vi "FFConstVI-Working.vi"(8 "nXForce":i32(slide) scale=-10000.0..10000.0, 11 "millisecond multiple":u32) -> ()   [LabVIEW 2013]
uses:
  FFConstdll/FFConstDll.dll
  user32.dll
panel:
  out "Acquire HRESULT":i32
  out "Current ForegroundWindow HWND":u32
  out "Start ForegroundWindow HWND":u32
  in  "stop":bool
  out "SetDeviceForce HRESULT":i32
  out "Init HRESULT":i32
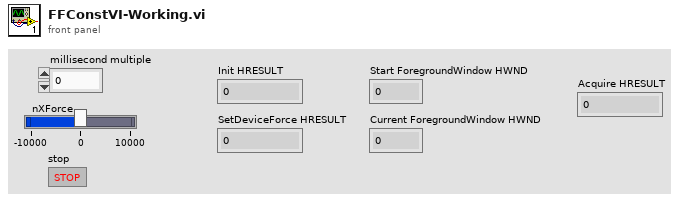
[diagram p1: front panel]
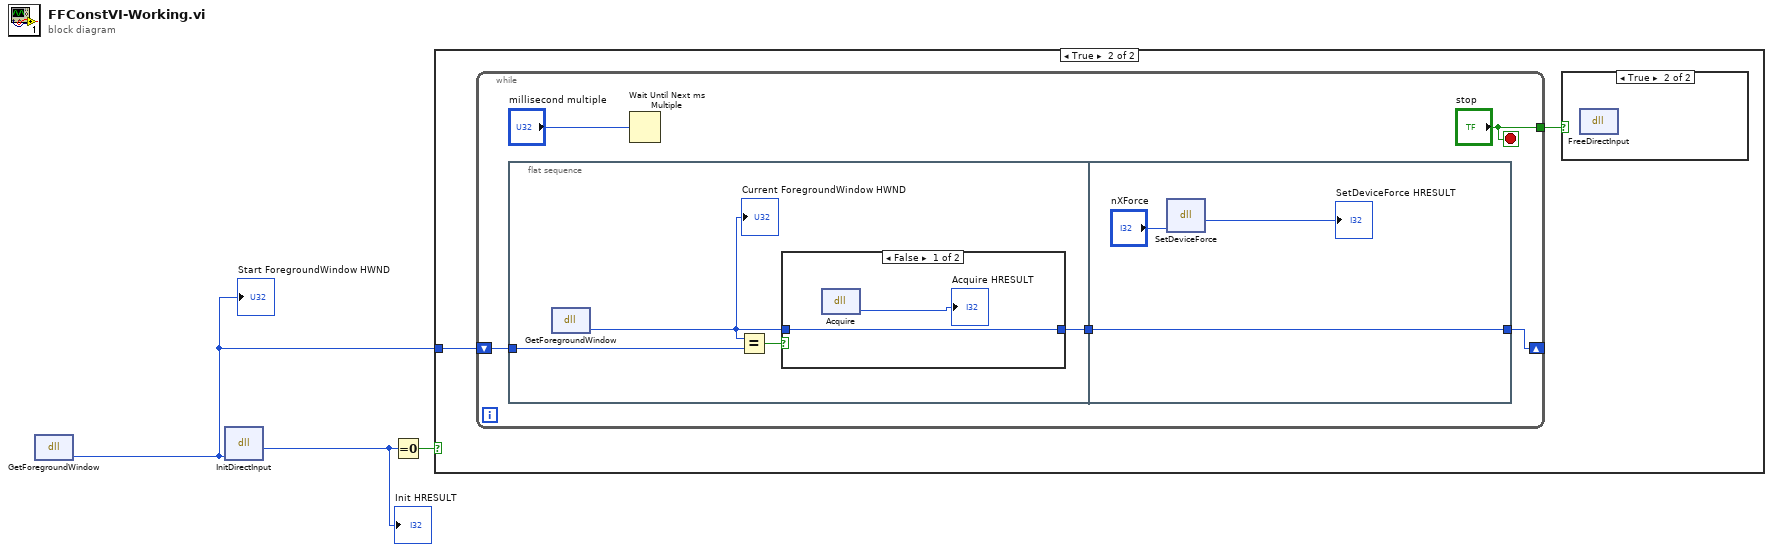
[diagram p0: block diagram]
diagram:
  n1 = dll-call lib="user32.dll" fn="GetForegroundWindow"() -> ("HWND"=w2:u32)  [unwired: 3 in, 2 out]
  "Start ForegroundWindow HWND" <- w2
  n2 = dll-call lib="C:/Users/user/Documents/Dropbox/Kettering/Robotics Team/RC Car Race Information/Teleop Labview Code/Winter '14 Force Feedback Experiment/FFConstdll/FFConstDll.dll" fn="InitDirectInput"("hDlg"=w2) -> ("HRESULT"=w1:u32)  [unwired: 4 in, 2 out]
  "Init HRESULT" <- w1
  n3 = Equal To 0?(x=w1) -> (x = 0?=w3:bool)
  n4 = case shown="True" w3 {
    tunnel: w2 -> [_ w4]
    frame False {
    }
    frame True {
      n5 = while {
        tunnel: ["stop"] -> w5
        shift-right: [w9] -> _
        shift-left: w4 -> [w7]
        stop <- "stop" stop-if-true
        n6 = flat-sequence {
          tunnel: w7 -> [w14]
          tunnel: [w11] -> w8
          tunnel: [w18] -> w9
          tunnel: w8 -> [w18]
          frame #0 {
            n7 = dll-call lib="user32.dll" fn="GetForegroundWindow"() -> ("HWND"=w12:u32)  [unwired: 3 in, 2 out]
            "Current ForegroundWindow HWND" <- w12
            n8 = Equal?(x=w12, y=w14) -> (x = y?=w13:bool)
            n9 = case shown="False" w13 {
              tunnel: w12 -> [w15 w17]
              tunnel: [w15 w17] -> w11
              frame False {
                n10 = dll-call lib="C:/Users/user/Documents/Dropbox/Kettering/Robotics Team/RC Car Race Information/Teleop Labview Code/Winter '14 Force Feedback Experiment/FFConstdll/FFConstDll.dll" fn="Acquire"() -> ("HRESULT"=→"Acquire HRESULT":i32)  [unwired: 3 in, 2 out]
              }
              frame True {
              }
            }
          }
          frame #1 {
            n11 = dll-call lib="C:/Users/user/Documents/Dropbox/Kettering/Robotics Team/RC Car Race Information/Teleop Labview Code/Winter '14 Force Feedback Experiment/FFConstdll/FFConstDll.dll" fn="SetDeviceForce"("nXForce"="nXForce") -> ("HRESULT"=→"SetDeviceForce HRESULT":i32)  [unwired: 4 in, 2 out]
          }
        }
        n12 = Wait Until Next ms Multiple(millisecond multiple="millisecond multiple") -> ()  [unwired: 1 out]
      }
      n13 = case shown="True" w5 {
        frame False {
        }
        frame True {
          n14 = dll-call lib="C:/Users/user/Documents/Dropbox/Kettering/Robotics Team/RC Car Race Information/Teleop Labview Code/Winter '14 Force Feedback Experiment/FFConstdll/FFConstDll.dll" fn="FreeDirectInput"() -> ()  [unwired: 4 in, 2 out]
        }
      }
    }
  }
